vi "Init.vi"(8 "error in (no error)":errorcluster, 11 "RHS_3D":refnum<class "NI_RHS_3D.lvclass">) -> (0 "error out":errorcluster, 3 "initialized RHS_3D":refnum<class "NI_RHS_3D.lvclass">)   [LabVIEW 2020, in "NI_PDE.lvlib" / "NI_RHS_3D.lvclass"]
uses:
  <vilib>/gmath/pde.llb/RHSClass/RHS_3D/NI_RHS_3D.lvclass
  <vilib>/gmath/pde.llb/RHSClass/Class Type.ctl
  <vilib>/gmath/pde.llb/RHSClass/NI_RHS.lvclass
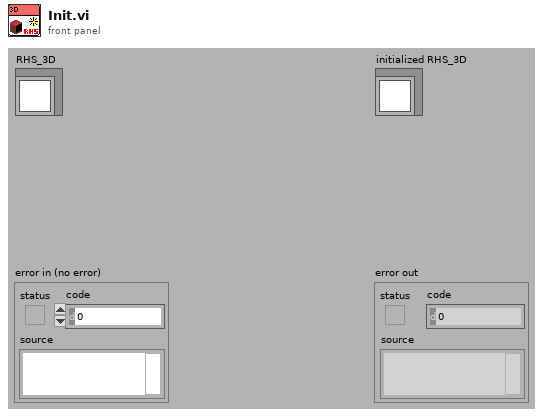
[diagram p1: front panel]
types:
  T1 = typedef "NI_PDE.lvlib/NI_RHS.lvclass/Class Type.ctl" = i32
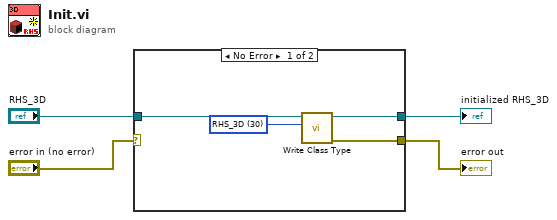
[diagram p0: block diagram]
diagram:
  n1 = case shown="No Error" "error in (no error)" {
    selector: "error in (no error)" -> [_ w10]
    tunnel: "RHS_3D" -> [w7 w9]
    tunnel: [w6 w9] -> w4
    tunnel: [w5 w10] -> w3
    frame No Error {
      w8 = T1 30 items=["RHS"=0, "RHS_2D"=20, "RHS_2D_Numeric"=21, "RHS_2D_VIRef"=22, "RHS_3D"=30, "RHS_3D_Numeric"=31, "RHS_3D_VIRef"=32] ("RHS class type")
      n2 = call-dynamic "Write Class Type.vi"("RHS class type"=w8, "RHS.lvclass in"=w7) -> ("error out"=w5:errorcluster, "RHS.lvclass out"=w6:refnum<class "NI_RHS_3D.lvclass">)  [unwired: 1 in, 7 out]
    }
    frame Error {
    }
  }
  "initialized RHS_3D" <- w4
  "error out" <- w3
